vi "LO_Reg.vi"(5 "Reg_Data":u32 format="%08x", 7 "RF":T3 items=["RF_0", "RF_1", "RF_2", "RF_3"], 8 "Error_In":errorcluster, 9 "LO":T1, 10 "RF_Ver":T2, 11 "VISA_Rsrc_In":refnum<visa-resource-name>) -> (0 "Error_Out":errorcluster, 3 "VISA_Rsrc_Out":refnum<visa-resource-name>)   [LabVIEW 2018]
uses:
  SP9500/Types/RF.ctl
  SP9500/Types/RF_Ver.ctl
  SP9500/Types/LO.ctl
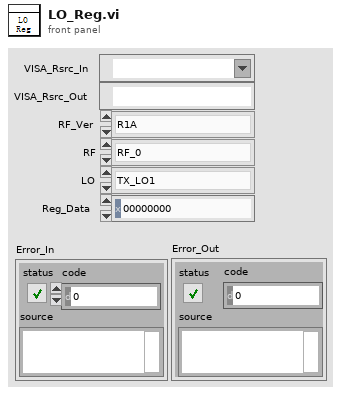
[diagram p1: front panel]
types:
  T1 = typedef "LO.ctl" = enum16{"TX_LO1", "TX_LO2", "TX_LO3", "RX_LO1", "RX_LO2", "RX_LO3"}
  T2 = typedef "RF_Ver.ctl" = enum16{"R1A", "R1B", "R1C", "R1D", "R1E", "R1F"}
  T3 = typedef "RF.ctl" = u16
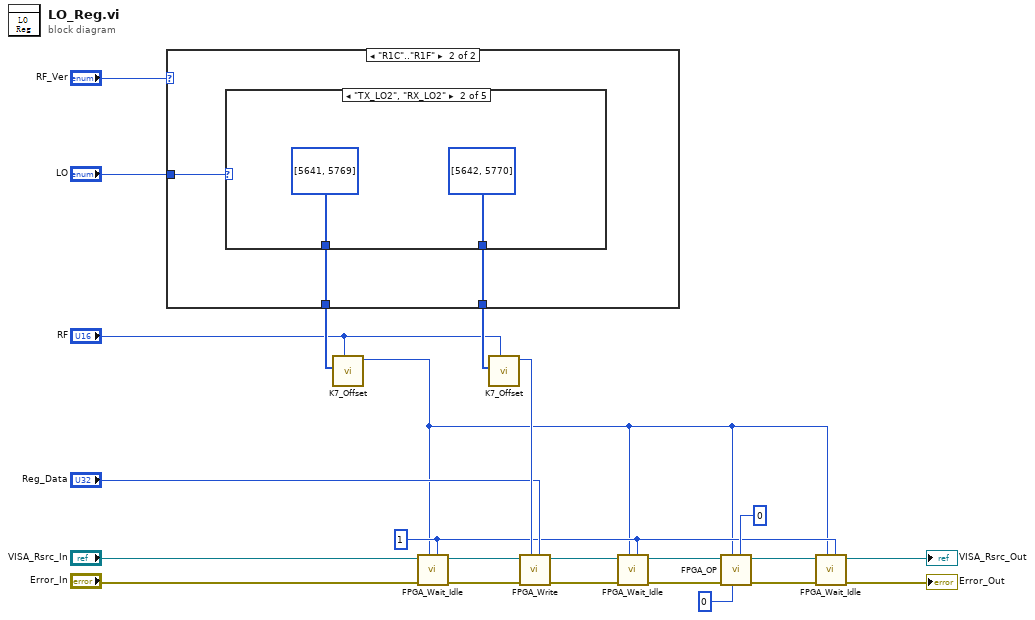
[diagram p0: block diagram]
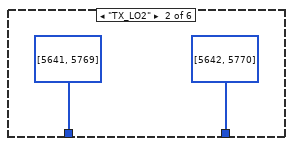
[diagram p3: hidden frame]
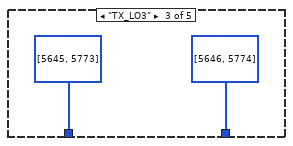
[diagram p9: hidden frame]
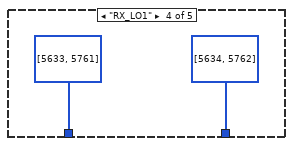
[diagram p10: hidden frame]
diagram:
  w6 = u32 1 ("Bit_Offset")
  n1 = case shown="\"R1C\"..\"R1F\"" "RF_Ver" {
    tunnel: "LO" -> [w26 w31]
    tunnel: [w25 w30] -> w21
    tunnel: [w24 w29] -> w20
    frame "R1A", "R1B" {
      n2 = case shown="\"TX_LO1\"" w26 {
        tunnel: [_ u32[] [5641, 5769] ("Offset") _ _ _ _] -> w25
        tunnel: [_ u32[] [5642, 5770] ("Offset") _ _ _ _] -> w24
        frame "TX_LO1" {
        }
        frame "TX_LO2" {
        }
        frame "TX_LO3" {
        }
        frame "RX_LO1" {
        }
        frame "RX_LO2" {
        }
        frame "RX_LO3" {
        }
      }
    }
    frame "R1C".."R1F" {
      n3 = case shown="\"TX_LO2\", \"RX_LO2\"" w31 {
        tunnel: [_ u32[] [5641, 5769] ("Offset") u32[] [5645, 5773] ("Offset") u32[] [5633, 5761] ("Offset") _] -> w30
        tunnel: [_ u32[] [5642, 5770] ("Offset") u32[] [5646, 5774] ("Offset") u32[] [5634, 5762] ("Offset") _] -> w29
        frame "TX_LO1" {
        }
        frame "TX_LO2", "RX_LO2" {
        }
        frame "TX_LO3" {
        }
        frame "RX_LO1" {
        }
        frame "RX_LO3" {
        }
      }
    }
  }
  n4 = call "K7_Offset.vi"("RF"="RF", "Offset"=w21) -> ("Offset"=w1:u32)  [unwired: 9 in]
  n5 = call "FPGA_Wait_Idle.vi"("Bit_Offset"=w6, "Offset"=w1, "Error_In"="Error_In", "VISA_Rsrc_In"="VISA_Rsrc_In") -> ("Error_Out"=w16:errorcluster, "VISA_Rsrc_Out"=w15:refnum<visa-resource-name>)  [unwired: 6 in]
  n6 = call "K7_Offset.vi"("RF"="RF", "Offset"=w20) -> ("Offset"=w18:u32)  [unwired: 9 in]
  n7 = call "FPGA_Write.vi"("Value"="Reg_Data", "Offset"=w18, "Error_In"=w16, "VISA_Rsrc_In"=w15) -> ("Error_Out"=w14:errorcluster, "VISA_Rsrc_Out"=w13:refnum<visa-resource-name>)  [unwired: 6 in]
  n8 = call "FPGA_Wait_Idle.vi"("Bit_Offset"=w6, "Offset"=w1, "Error_In"=w14, "VISA_Rsrc_In"=w13) -> ("Error_Out"=w11:errorcluster, "VISA_Rsrc_Out"=w12:refnum<visa-resource-name>)  [unwired: 6 in]
  n9 = call "FPGA_OP.vi"("Origin_Value"=u32 0, "OP_Offset"=u32 0, "Offset"=w1, "Error_In"=w11, "VISA_Rsrc_In"=w12) -> ("Error_Out"=w7:errorcluster, "VISA_Rsrc_Out"=w8:refnum<visa-resource-name>)  [unwired: 5 in]
  n10 = call "FPGA_Wait_Idle.vi"("Bit_Offset"=w6, "Offset"=w1, "Error_In"=w7, "VISA_Rsrc_In"=w8) -> ("Error_Out"=→"Error_Out":errorcluster, "VISA_Rsrc_Out"=→"VISA_Rsrc_Out":refnum<visa-resource-name>)  [unwired: 6 in]
